vi "Material-UnLoad-ResultCheck.vi"(8 "error in (no error)":errorcluster, 11 "Material-RunTest in":refnum<class "Material-RunTest.lvclass">) -> (0 "error out":errorcluster, 3 "Material-RunTest out":refnum<class "Material-RunTest.lvclass">)   [LabVIEW 2014, in "Material-RunTest.lvclass"]
uses:
  Material-RunTest.lvclass
  Material-RunTest.lvclass/Material-RunTest.ctl
  <userlib>/_OpenG.lib/array/array.llb/Search 1D Array (Boolean)__ogtk.vi
  <userlib>/_OpenG.lib/array/array.llb/Empty 1D Array (I32)__ogtk.vi
  ITS-FlexMotion/FlexMotion_Control.lvclass
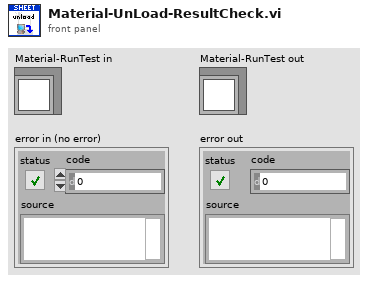
[diagram p1: front panel]
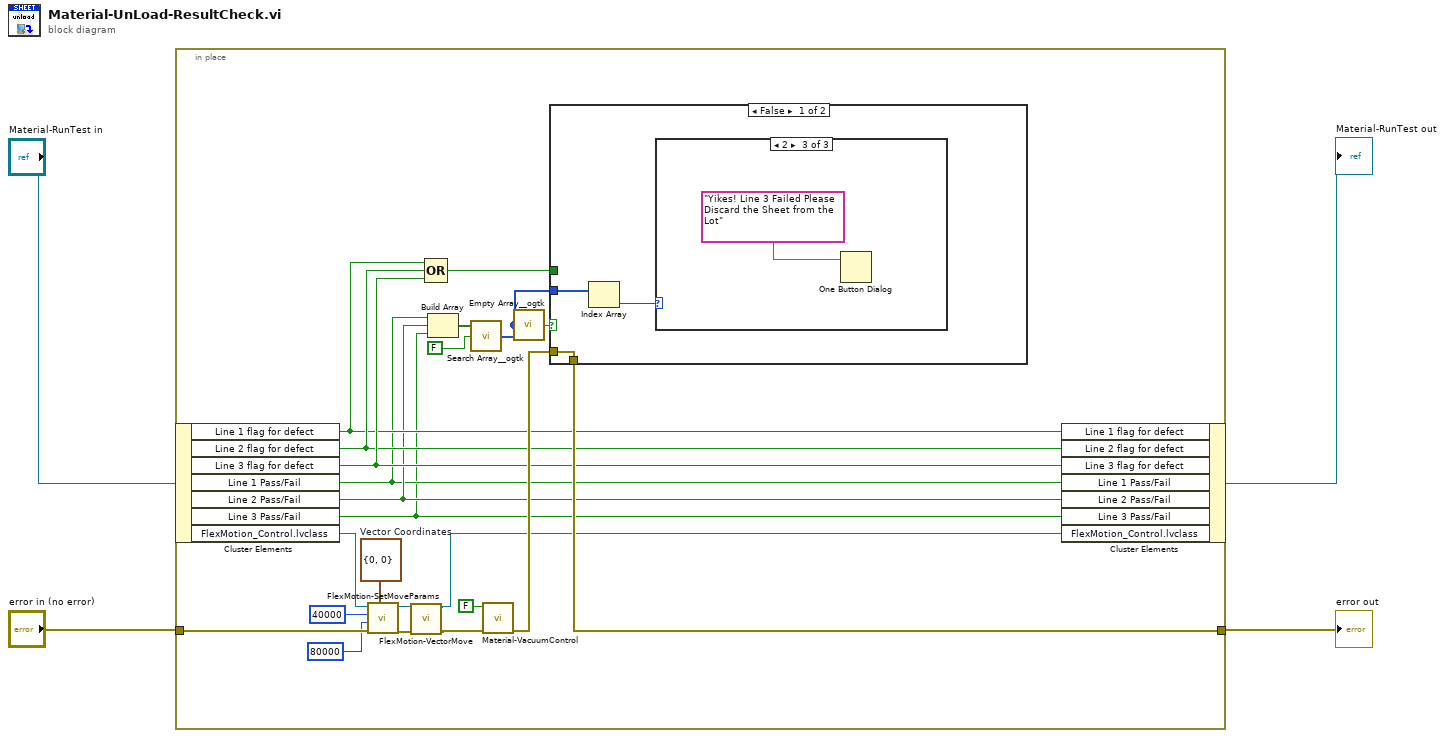
[diagram p0: block diagram]
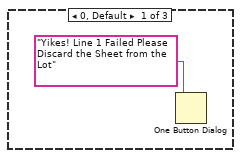
[diagram p2: hidden frame]
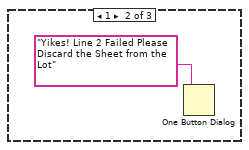
[diagram p3: hidden frame]
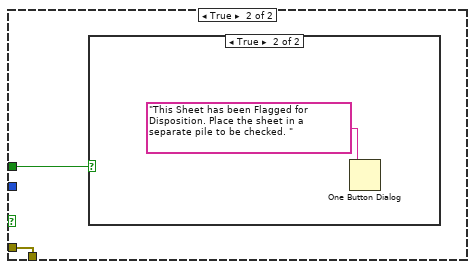
[diagram p4: hidden frame]
diagram:
  n1 = in-place {
    in-place-border: "error in (no error)" -> [w13]
    in-place-border: [w25] -> w3
    w7 = cluster{"X Position":i32, "Y Position":i32} {"X Position"=0, "Y Position"=0}  # Vector Coordinates
    n2 = in-place-cluster #1("Material-RunTest in") -> ("Line 1 flag for defect"=w22:bool, "Line 2 flag for defect"=w23:bool, "Line 3 flag for defect"=w24:bool, "Line 1 Pass/Fail"=w19:bool, "Line 2 Pass/Fail"=w20:bool, "Line 3 Pass/Fail"=w18:bool, "FlexMotion_Control.lvclass"=w12:refnum<class "FlexMotion_Control.lvclass">)
    n3 = call "FlexMotion-SetMoveParams.vi"("Vector Coordinates"=w7, "error in"=w13, "Acceleration"=u32 80000, "Velocity"=40000, "FlexMotion_Control.lvclass"=w12) -> ("error out"=w11:errorcluster, "FlexMotion_Control.lvclass"=w8:refnum<class "FlexMotion_Control.lvclass">)  [unwired: 5 in]
    n4 = call "FlexMotion-VectorMove.vi"("error in"=w11, "FlexMotion_Control.lvclass"=w8) -> ("error out"=w10:errorcluster, "FlexMotion_Control.lvclass"=w9:refnum<class "FlexMotion_Control.lvclass">)  [unwired: 8 in]
    n5 = Compound Arithmetic op=OR(w22, w23, w24) -> (w21:bool)
    n6 = Build Array(w19, w20, w18) -> (w17:bool[])
    n7 = call-poly <userlib>:"Search Array__ogtk.vi"("Array"=w17, "Element Data"=FALSE) -> ("Indices of Elements"=w14:i32[])  [unwired: 7 in]
    n8 = call "Material-VacuumControl.vi"("error in (no error)"=w10, "Vacuum On/Off"=FALSE) -> ("error out"=w26:errorcluster)  [unwired: 9 in]
    n9 = call-poly <userlib>:"Empty Array__ogtk.vi"("Array"=w14) -> ("Empty Array?"=w15:bool)  [unwired: 8 in]
    n10 = case shown="False" w15 {
      tunnel: w26 -> [w30 w35]
      tunnel: [w30 w35] -> w25
      tunnel: w21 -> [_ w34]
      tunnel: w14 -> [w29 _]
      frame False {
        n11 = Index Array(array=w29) -> (element=w28:i32)  [unwired: 1 in]
        n12 = case shown="2" w28 {
          frame 0, Default {
            n13 = One Button Dialog(message="Yikes! Line 1 Failed Please Discard the Sheet from the Lot") -> ()  [unwired: 1 in, 1 out]
          }
          frame 1 {
            n14 = One Button Dialog(message="Yikes! Line 2 Failed Please Discard the Sheet from the Lot") -> ()  [unwired: 1 in, 1 out]
          }
          frame 2 {
            n15 = One Button Dialog(message="Yikes! Line 3 Failed Please Discard the Sheet from the Lot") -> ()  [unwired: 1 in, 1 out]
          }
        }
      }
      frame True {
        n16 = case shown="True" w34 {
          frame False {
          }
          frame True {
            n17 = One Button Dialog(message="This Sheet has been Flagged for Disposition. Place the sheet in a separate pile to be checked. ") -> ()  [unwired: 1 in, 1 out]
          }
        }
      }
    }
    n18 = in-place-cluster #1("Line 1 flag for defect"=w22, "Line 2 flag for defect"=w23, "Line 3 flag for defect"=w24, "Line 1 Pass/Fail"=w19, "Line 2 Pass/Fail"=w20, "Line 3 Pass/Fail"=w18, "FlexMotion_Control.lvclass"=w9) -> (→"Material-RunTest out":refnum<class "Material-RunTest.lvclass">)
  }
  "error out" <- w3
